vi "MPU-6050 Gyro & Accelrometer using Arduino .vi"() -> ()   [LabVIEW 2020]
uses:
  <vilib>/MakerHub/LINX/Public/Sensors/Accelerometer/MPU60X0/DeviceAddresses.ctl
  <vilib>/MakerHub/LINX/Public/Utilities/Open Serial.vi
  <vilib>/MakerHub/LINX/Public/Sensors/Accelerometer/MPU60X0/MPU60X0.lvlib
  <vilib>/MakerHub/LINX/LMH-LINX.lvlib
panel:
  out "Gyro (degree / sec)":T1(graph)
  out "Acceleration (g)":T1(graph)
  out "3D Picture":refnum<vi>(3d-picture)
  out "Acceleration Data (g)":T1
  out "Gyro  Data (dps)":T1
  in  "stop":bool
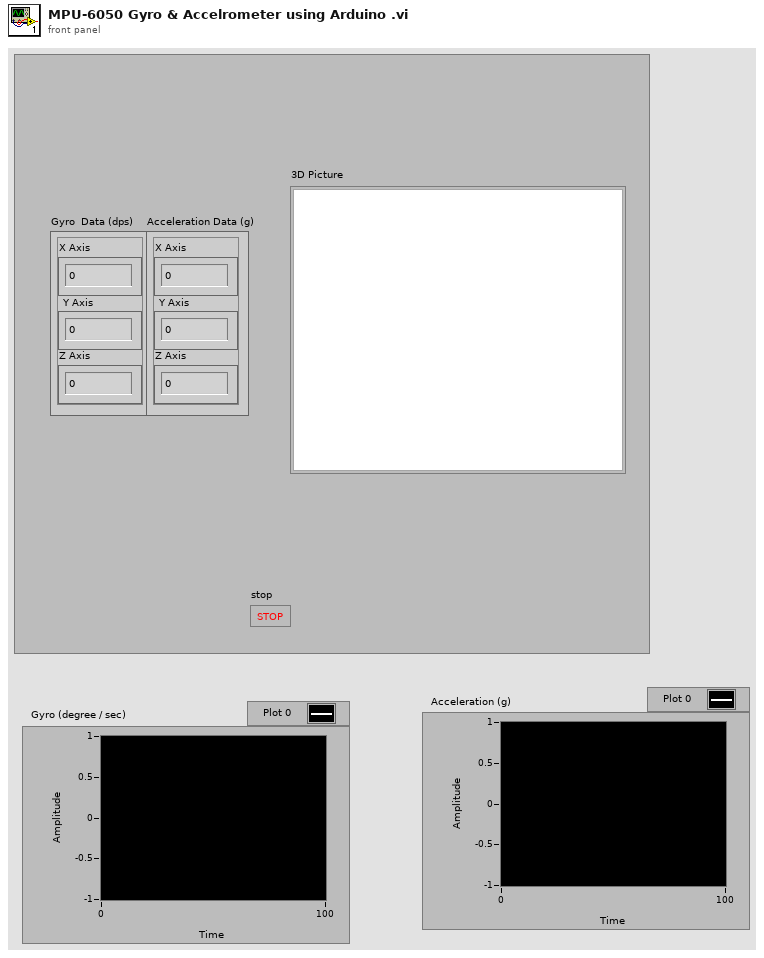
[diagram p1: front panel]
types:
  T1 = cluster{"X Axis":i16, "Y Axis":i16, "Z Axis":i16}
  T2 = typedef "LMH-LINX.lvlib/MPU60X0.lvlib/DeviceAddresses.ctl" = enum16{"0x68", "0x69"}
  T3 = typedef "LMH-LINX.lvlib/LINX Ref.ctl" = cluster{"IO":T4, "Interface":T5, "LINX Device Config":T6}
  T4 = typedef "LMH-LINX.lvlib/Platform.ctl" = enum16{"Remote", "Local"}
  T5 = typedef "LMH-LINX.lvlib/Interface.ctl" = enum16{"Serial", "TCP"}
  T6 = typedef "LMH-LINX.lvlib/Device.lvlib/LINX Device Config.ctl" = cluster{"Interface":T5, "COM Port":refnum<visa-resource-name>, "TCP Configuration":T7, "Device Family":u8, "Device ID":u8, "Device Name":string, "TCP Ref":refnum<k5>, "Channels":T8}
  T7 = typedef "LMH-LINX.lvlib/Device.lvlib/TCP Config.ctl" = cluster{"IP Address":string, "Port":u16}
  T8 = typedef "LMH-LINX.lvlib/Channels.ctl" = cluster{"DI":u8[], "DO":u8[], "AI":u8[], "AO":u8[], "PWM":u8[], "QE":u8[], "UART":u8[], "I2C 2":u8[], "SPI":u8[], "CAN":u8[], "Servo":u8[], "AI Ref (V)":dbl, "AI Resolution (Bits)":u8, "AO Ref (V)":dbl, "AO Resolution (Bits)":u8}
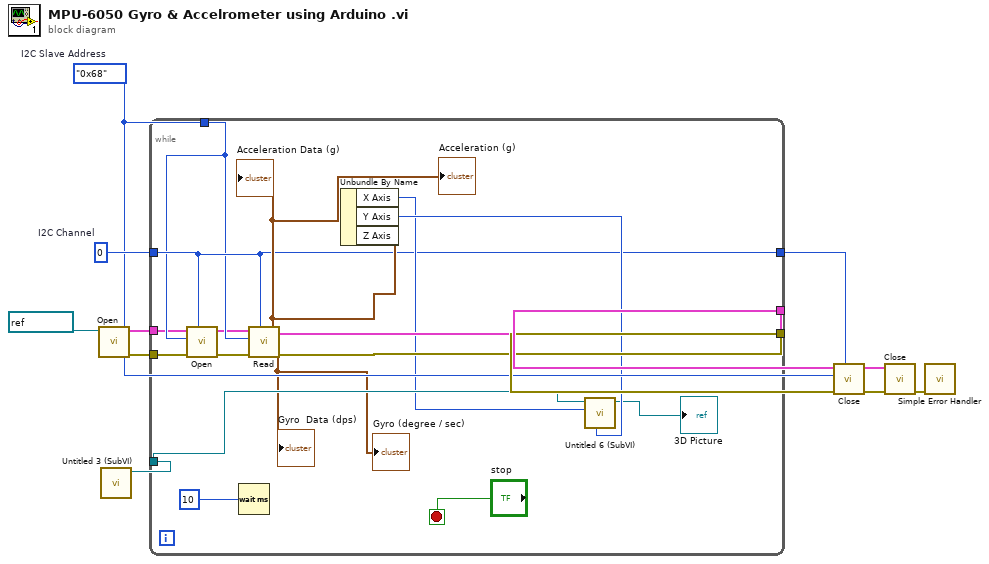
[diagram p0: block diagram]
diagram:
  w7 = u8 0  # I2C Channel
  w2 = DeviceAddresses."0x68"  # I2C Slave Address
  n1 = call-poly <vilib>:"Open.vi"("Serial Port"=refnum<visa-resource-name> "COM3") -> ("Error Out"=w3:errorcluster, "LINX Resource"=w1:T3)  [unwired: 8 in, 1 out]
  n2 = call "Untitled 3 (SubVI).vi"() -> ("SceneObject out"=w4:refnum<vi>)  [unwired: 11 in]
  n3 = while {
    tunnel: [w28] -> w11
    tunnel: [w27] -> w10
    tunnel: w7 -> [w19]
    tunnel: [w19] -> w6
    tunnel: w4 -> [w25]
    tunnel: w3 -> [w18]
    tunnel: w2 -> [w17]
    tunnel: w1 -> [w16]
    stop <- "stop" stop-if-true
    n4 = call <vilib>:"Open.vi"("I2C Channel"=w19, "Error In"=w18, "I2C Slave Address"=w17, "LINX Resource"=w16) -> ("Error Out"=w15:errorcluster, "LINX Resource"=w14:T3)  [unwired: 6 in]
    n5 = Wait (ms)(milliseconds to wait=u32 10) -> ()  [unwired: 1 out]
    n6 = call <vilib>:"Read.vi"("I2C Channel"=w19, "Error In"=w15, "I2C Slave Address"=w17, "LINX Resource"=w14) -> ("Error Out"=w27:errorcluster, "Gyro  Data (dps)"=→"Gyro  Data (dps)" →"Gyro (degree / sec)":T1, "Acceleration Data (g)"=w21:T1, "LINX Resource"=w28:T3)  [unwired: 3 in, 1 out]
    "Acceleration Data (g)" <- w21
    "Acceleration (g)" <- w21
    n7 = Unbundle By Name(w21) -> ("X Axis"=w22:i16, "Y Axis"=w24:i16)  [unwired: 1 out]
    n8 = call "Untitled 6 (SubVI).vi"("Angle Y"=w24, "Angle X"=w22, "SceneObject in"=w25) -> ("SceneObject out"=→"3D Picture":refnum<vi>)  [unwired: 8 in]
  }
  n9 = call <vilib>:"Close.vi"("I2C Channel (0)"=w6, "Error In"=w10, "I2C Slave Address (0)"=w2, "LINX Resource"=w11) -> ("Error Out"=w9:errorcluster, "LINX Resource"=w12:T3)  [unwired: 6 in]
  n10 = call <vilib>:"Close.vi"("Error In"=w9, "LINX Resource"=w12) -> ("Error Out"=w8:errorcluster)  [unwired: 9 in]
  n11 = call <vilib>:"Simple Error Handler.vi"("error in (no error)"=w8) -> ()  [unwired: 4 in, 5 out]
